vi "全局 3.vi"() -> ()   [LabVIEW 2016]
panel:
  in  "布尔":bool
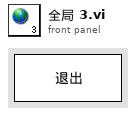
[diagram p1: front panel]
diagram:
